vi "Get First Matched Node.vi"(8 "error in (no error)":errorcluster, 10 "XPath expression":string, 11 "node in":refnum<k20>) -> (0 "error out":errorcluster, 2 "node result":refnum<k20>, 3 "node out":refnum<k20>)   [LabVIEW 2020, in "NI_XML.lvlib"]
doc: "Returns the first node within <B>node in</B> that matches the <B>XPath expression</B>. If this VI does not find a match, <B>node result</B> is not a valid refnum."
uses:
  <vilib>/xml/NI_XML.lvlib
  DOMUserDefRef.dll
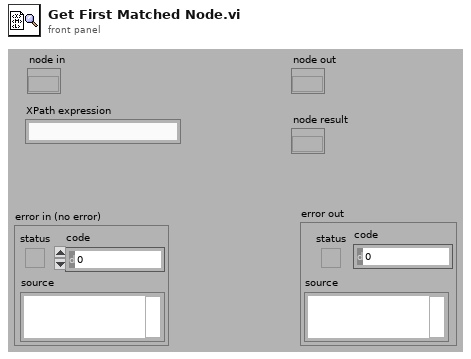
[diagram p1: front panel]
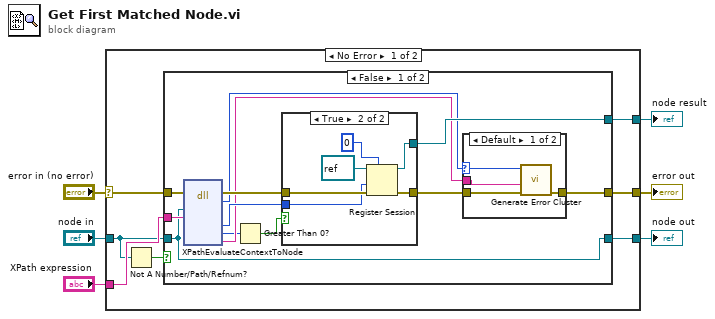
[diagram p0: block diagram]
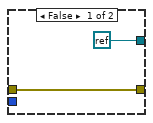
[diagram p2: hidden frame]
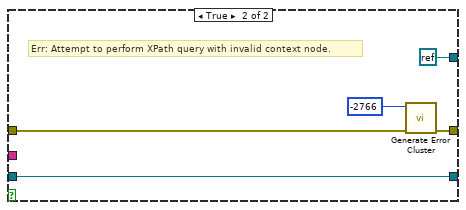
[diagram p4: hidden frame]
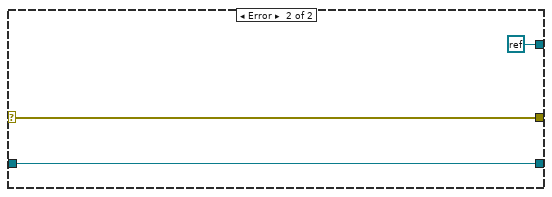
[diagram p5: hidden frame]
diagram:
  n1 = case shown="No Error" "error in (no error)" {
    selector: "error in (no error)" -> [w7 w46]
    tunnel: "XPath expression" -> [w13 _]
    tunnel: [w12 refnum<k0> refnum ("Not a Refnum Constant")] -> w5
    tunnel: [w11 w46] -> w4
    tunnel: [w10 w45] -> w3
    tunnel: "node in" -> [w8 w45]
    frame No Error {
      n2 = Not A Number/Path/Refnum?(number/path/refnum=w8) -> (NaN/Path/Refnum?=w9:bool)
      n3 = case shown="False" w9 {
        tunnel: w13 -> [w25 _]
        tunnel: [w22 refnum<k0> refnum ("Not a Refnum Constant")] -> w12
        tunnel: [w20 w40] -> w11
        tunnel: [w17 w43] -> w10
        tunnel: w8 -> [w17 w43]
        tunnel: w7 -> [w14 w41]
        frame False {
          n4 = dll-call lib="DOMUserDefRef.*" fn="XPathEvaluateContextToNode"(error in=w14, "session"=w17, "xpathStr"=w25) -> (error out=w24:errorcluster, "retErr"=w15:i32, "retSess"=w23:u64, "numNodes"=w16:u32, "errIOString"=w19:string)  [unwired: 3 in, 5 out]
          n5 = Greater Than 0?(x=w16) -> (x > 0?=w18:bool)
          n6 = case shown="True" w18 {
            tunnel: w24 -> [w27 w32]
            tunnel: w23 -> [_ w30]
            tunnel: [refnum<k0> refnum ("Not a Refnum Constant") w29] -> w22
            tunnel: [w27 w28] -> w21
            frame False {
            }
            frame True {
              n7 = Register Session(7:0 ("cleanup mode (default to class = 0)"), 8:w32, 9:w30, 11:refnum<k20> refnum ("Node Reg")) -> (0:w28:errorcluster, 3:w29:refnum<k20>)  [unwired: 1 in]
            }
          }
          n8 = case shown="Default" w15 {
            selector: w15 -> [w37 _]
            tunnel: w19 -> [w36 _]
            tunnel: w21 -> [w35 w38]
            tunnel: [w34 w38] -> w20
            frame Default {
              n9 = call <vilib>:"Generate Error Cluster.vi"("error in (no error)"=w35, "Additional Message"=w36, "Code"=w37) -> ("error out"=w34:errorcluster)  [unwired: 8 out]
            }
            frame 0 {
              # "No Error"
            }
          }
        }
        frame True {
          # "Err: Attempt to perform XPath query with invalid context node."
          n10 = call <vilib>:"Generate Error Cluster.vi"("error in (no error)"=w41, "Code"=-2766) -> ("error out"=w40:errorcluster)  [unwired: 1 in, 8 out]
        }
      }
    }
    frame Error {
    }
  }
  "error out" <- w4
  "node out" <- w3
  "node result" <- w5
